vi "Inherits from an Actor.vi"(7 "App Reference (this app)":refnum<vi>, 8 "error in (no error)":errorcluster, 11 "Path":path) -> (0 "error out":errorcluster, 1 "Default Actor Path":path, 2 "Is Path to Actor?":bool)   [LabVIEW 2021, in "Message Maker.lvlib"]
uses:
  Message Maker.lvlib
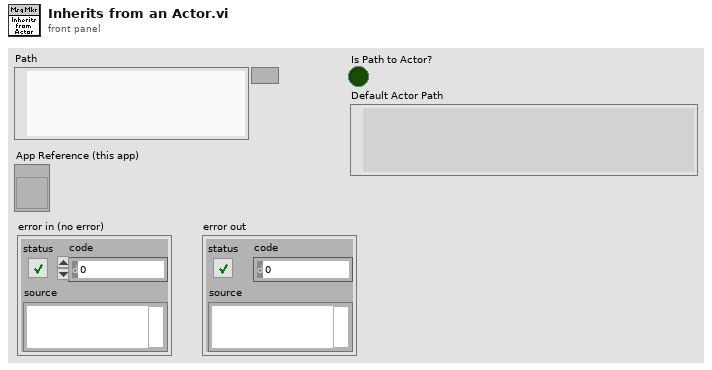
[diagram p1: front panel]
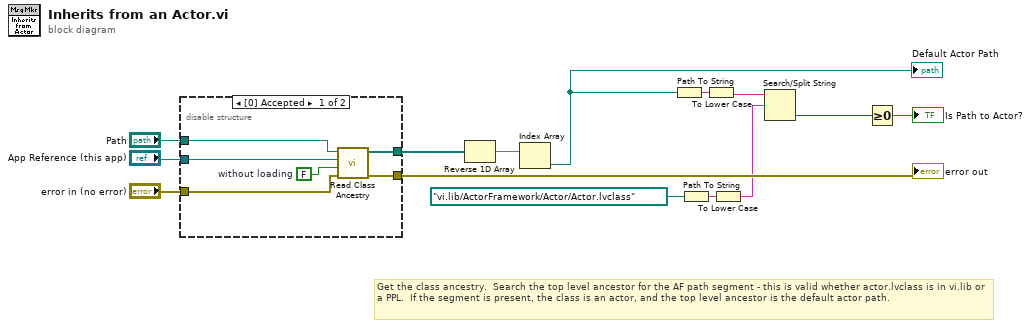
[diagram p0: block diagram]
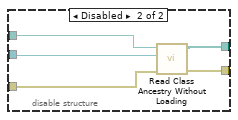
[diagram p2: hidden frame]
diagram:
  # "Get the class ancestry.  Search the top level ancestor for the AF path segment - this is valid whether actor.lvclass is in vi.lib or a PPL.  If the segment is present, the class is an actor, and the top level ancestor is the default actor path."
  n1 = disable-structure shown="[0] Accepted" {
    disable-tunnel: [w20 w25] -> w14
    disable-tunnel: "Path" -> [w19 w23]
    disable-tunnel: "error in (no error)" -> [w18 w22]
    disable-tunnel: [w17 w24] -> w8
    disable-tunnel: "App Reference (this app)" -> [w16 w21]
    frame Enabled {
      w15 = FALSE  # without loading
      n2 = call <vilib>:"Read Class Ancestry.vi"("error in (no error)"=w18, "without loading"=w15, "App Reference (this app)"=w16, "LabVIEW Class Path"=w19) -> ("error out"=w20:errorcluster, "Class Ancestry"=w17:path[])  [unwired: 6 in]
    }
    frame Disabled {
      n3 = call <vilib>:"Read Class Ancestry Without Loading.vi"("error in (no error)"=w22, "App Reference (this app)"=w21, "LabVIEW Class Path"=w23) -> ("error out"=w25:errorcluster, "Class Ancestry"=w24:path[])  [unwired: 7 in]
    }
  }
  "error out" <- w14
  n4 = Reverse 1D Array(array=w8) -> (reversed array=w7:path[])
  n5 = Index Array(array=w7) -> (element=w9:path)  [unwired: 1 in]
  "Default Actor Path" <- w9
  n6 = Path To String(path=w9) -> (string=w5:string)
  n7 = Path To String(path=path "vi.lib/ActorFramework/Actor/Actor.lvclass") -> (string=w4:string)
  n8 = To Lower Case(string=w5) -> (all lower case string=w3:string)
  n9 = To Lower Case(string=w4) -> (all lower case string=w2:string)
  n10 = Search/Split String(string=w3, search string/char (-)=w2) -> (offset of match=w13:i32)  [unwired: 1 in, 2 out]
  n11 = Greater Or Equal To 0?(x=w13) -> (x >= 0?=→"Is Path to Actor?":bool)
